vi "MTSS-masny.vi"(1 "scale":dbl=1.0 min=1.0, 2 "h":dbl, 3 "frame size":cluster{"frame-x":dbl, "frame-y":dbl}) -> (0 "Pic out":picture)   [LabVIEW 2019]
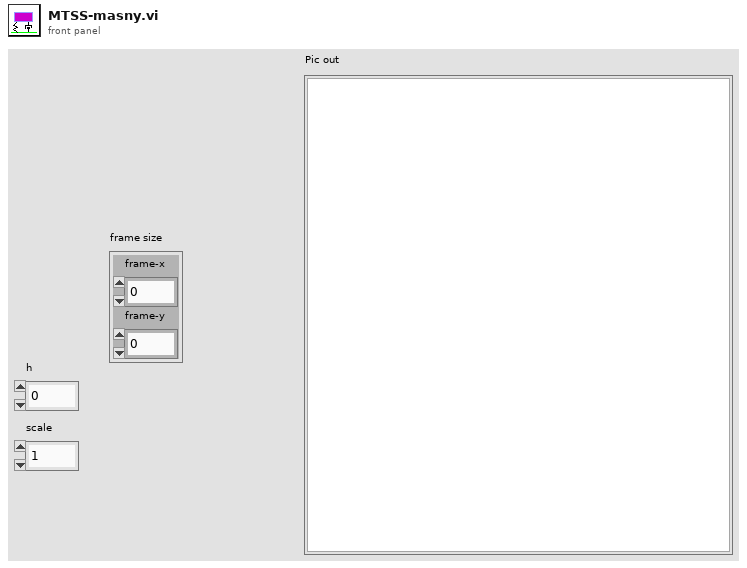
[diagram p1: front panel]
types:
  T1 = cluster{"Width":u16, "Style":enum32{"Solid", "Dash", "Dot", "DashDot", "DashDotDot"}}
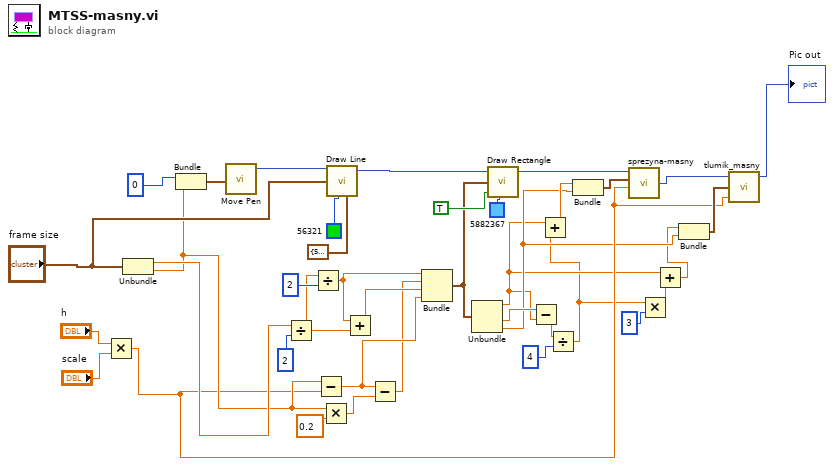
[diagram p0: block diagram]
diagram:
  n1 = Multiply(x="h", y="scale") -> (x*y=w8:dbl)
  n2 = Unbundle("frame size") -> ("frame-x"=w29:dbl, "frame-y"=w21:dbl)
  n3 = Bundle(0, "frame-y"=w21) -> (w39:cluster{i32, "frame-y":dbl})  [unwired: 1 in]
  n4 = call <vilib>:"Move Pen.vi"("new position"=w39) -> ("new picture"=w38:picture)  [unwired: 4 in]
  n5 = Divide(x=w29, y=2) -> (x/y=w25:dbl)
  n6 = Divide(x=w25, y=2) -> (x/y=w24:dbl)
  n7 = Subtract(x=w21, y=w8) -> (x-y=w19:dbl)
  n8 = Multiply(x=w21, y=0.2) -> (x*y=w20:dbl)
  n9 = call <vilib>:"Draw Line.vi"("picture"=w38, "end point"="frame size", "color(black)"=u32 56321, "pen"=T1 {"Width"=5, "Style"=enum."Solid"}) -> ("new picture"=w31:picture)  [unwired: 5 in]
  n10 = Add(x=w24, y=w25) -> (x+y=w23:dbl)
  n11 = Subtract(x=w19, y=w20) -> (x-y=w18:dbl)
  n12 = Bundle(w24, w18, w23, w19) -> (w16:cluster{dbl, dbl, dbl, dbl})  [unwired: 1 in]
  n13 = Unbundle(w16) -> (w5:dbl, w12:dbl, w6:dbl)  [unwired: 1 out]
  n14 = call <vilib>:"Draw Rectangle.vi"("picture"=w31, "rect"=w16, "fill?(F)"=TRUE, "color(black)"=u32 5882367) -> ("new picture"=w17:picture)  [unwired: 5 in]
  n15 = Subtract(x=w12, y=w5) -> (x-y=w15:dbl)
  n16 = Divide(x=w15, y=4) -> (x/y=w3:dbl)
  n17 = Add(x=w5, y=w3) -> (x+y=w10:dbl)
  n18 = Bundle(w10, w6) -> (w13:cluster{dbl, dbl})  [unwired: 1 in]
  n19 = call "sprezyna-masny.vi"("h"=w8, "x0y0"=w13, "Pic in"=w17) -> ("Pic out"=w11:picture)  [unwired: 3 in]
  n20 = Multiply(x=w3, y=3) -> (x*y=w2:dbl)
  n21 = Add(x=w5, y=w2) -> (x+y=w1:dbl)
  n22 = Bundle(w1, w6) -> (w9:cluster{dbl, dbl})  [unwired: 1 in]
  n23 = call "tlumik_masny.vi"("h"=w8, "x0y0"=w9, "Pic in"=w11) -> ("Pic out"=→"Pic out":picture)  [unwired: 2 in]
